vi "Unflatten-MouseMotionEventData.vi"(8 "error in (no error)":errorcluster, 11 "Event Binary Data":string) -> (0 "error out":errorcluster, 3 "MouseMotionEvent":T1 {"State" items=["SDL_BUTTON_LEFT"=1, "SDL_BUTTON_MIDDLE"=2, "SDL_BUTTON_RIGHT"=3, "SDL_BUTTON_X1"=4, "SDL_BUTTON_X2"=5]})   [LabVIEW 2026, in "SDL3.lvlib" / "Events.lvlib"]
uses:
  Events.lvlib
  MouseMotionEvent--cluster.ctl
  Video/WindowID--integer.ctl
  Mouse/MouseID--integer.ctl
  Mouse/MouseButtonFlags--ring.ctl
  Video/Video.lvlib
  Mouse/Mouse.lvlib
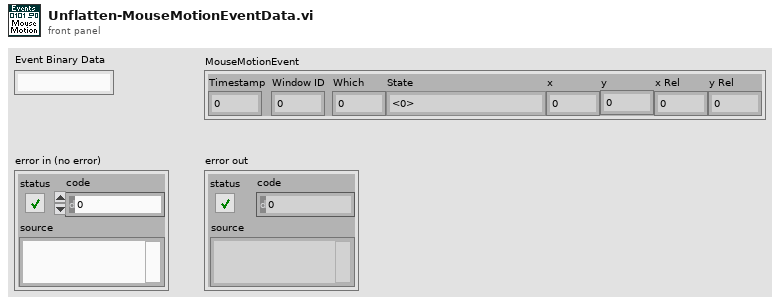
[diagram p1: front panel]
types:
  T1 = typedef "SDL3.lvlib/Events.lvlib/MouseMotionEvent--cluster.ctl" = cluster{"Timestamp":u64, "Window ID":T2, "Which":T3, "State":T4, "x":sgl, "y":sgl, "x Rel":sgl, "y Rel":sgl}
  T2 = typedef "SDL3.lvlib/Video.lvlib/WindowID--integer.ctl" = u32
  T3 = typedef "SDL3.lvlib/Mouse.lvlib/MouseID--integer.ctl" = u32
  T4 = typedef "SDL3.lvlib/Mouse.lvlib/MouseButtonFlags--ring.ctl" = u32
  T5 = enum16{"big-endian, network order", "native, host order", "little-endian"}
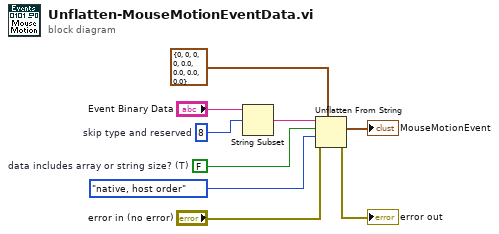
[diagram p0: block diagram]
diagram:
  w2 = 8  # skip type and reserved
  w6 = FALSE  # data includes array or string size? (T)
  n1 = String Subset(string="Event Binary Data", offset (0)=w2) -> (substring=w3:string)  [unwired: 1 in]
  n2 = Unflatten From String(type=T1 {"Timestamp"=0, "Window ID"=0, "Which"=0, "State"=0, "x"=0.0, "y"=0.0, "x Rel"=0.0, "y Rel"=0.0} ("MouseMotionEvent"), binary string=w3, data includes array or string size? (T)=w6, byte order (0:big-endian, network order)=T5."native, host order", error in (no error)="error in (no error)") -> (value=→"MouseMotionEvent":T1, error out=→"error out":errorcluster)  [unwired: 1 out]
